vi "Connect.vi"(8 "error in (no error)":errorcluster, 11 "336XX in":refnum<class "336XX.lvclass">) -> (0 "error out":errorcluster, 3 "336XX out":refnum<class "336XX.lvclass">)   [LabVIEW 2019, in "336XX.lvlib" / "336XX.lvclass"]
uses:
  Library/336XX.lvclass
  C:/Users/Public/Documents/Development/builds/Instruments/Instruments.lvlibp/Library/Instruments.lvclass
  Library/336XX.lvclass/336XX.ctl
  builds/Instruments/Instruments.lvlibp/Accessors/Read Resource.vi
  builds/Instruments/FunctionGenerator.lvlibp/Library/FunctionGenerator.lvclass
  <instrlib>/Agilent 3352X Series/Agilent 3352X Series.lvlib
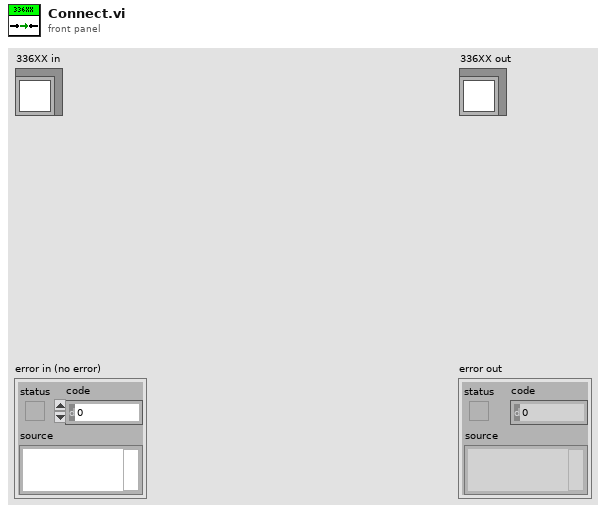
[diagram p1: front panel]
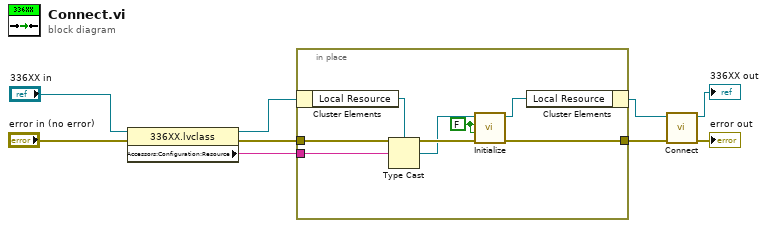
[diagram p0: block diagram]
diagram:
  n1 = property class="336XX.lvclass"(reference="336XX in", error in="error in (no error)") -> (reference out=w5:refnum<class "336XX.lvclass">, error out=w4:errorcluster, "Accessors:Configuration:Resource"=w3:string)
  n2 = in-place {
    in-place-border: w4 -> [w16]
    in-place-border: w3 -> [w12]
    in-place-border: [w15] -> w2
    w10 = FALSE ("ID Query (Enable)")
    n3 = in-place-cluster #1(w5) -> ("Local Resource"=w13:refnum<visa-resource-name>)
    n4 = Type Cast(type=w13, x=w12) -> (*(type *) &x=w11:refnum<visa-resource-name>)
    n5 = call <instrlib>:"Initialize.vi"("error in (no error)"=w16, "Reset (Enable)"=w10, "ID Query (Enable)"=w10, "VISA resource name"=w11) -> ("error out"=w15:errorcluster, "VISA resource name out"=w14:refnum<visa-resource-name>)  [unwired: 6 in]
    n6 = in-place-cluster #1("Local Resource"=w14) -> (w1:refnum<class "336XX.lvclass">)
  }
  n7 = call-parent "Connect.vi"("error in (no error)"=w2, "FunctionGenerator in"=w1) -> ("error out"=→"error out":errorcluster, "FunctionGenerator out"=→"336XX out":refnum<class "336XX.lvclass">)  [unwired: 8 in]
